vi "test(Subvi).vi"(6 "Frequency(Hz)":dbl, 8 "Amplitude(Vpeak)":dbl, 9 "Pulse length(sec)":dbl, 10 "Delay time.A.1(sec)":dbl, 11 "Sampling frequency(Hz)":dbl) -> ()   [LabVIEW 2017]
uses:
  <vilib>/Analysis/3filter.llb/Filter Passband Type.ctl
  <vilib>/Analysis/4window.llb/windowTd.ctl
  <vilib>/measure/maspectr.llb/FFT Spectrum (Real-Im) for 1 Chan.vi
  <vilib>/Analysis/3filter.llb/FIR Windowed Filter (DBL).vi
  <vilib>/Analysis/NI_AALBase.lvlib
  <vilib>/measure/NI_MAPro.lvlib
  <vilib>/Analysis/NI_AALPro.lvlib
panel:
  out "웨이브폼 그래프 7":waveform(dbl)(graph)
  out "웨이브폼 그래프 6":waveform(dbl)(graph)
  out "웨이브폼 그래프 3":dbl[](graph)
  out "크기":i32
  in  "Carrier Frequency(Hz)":dbl
  out "Delay SIG.A.1":dbl[](array[numeric])
  out "Pulse SIG":dbl[](array[numeric])
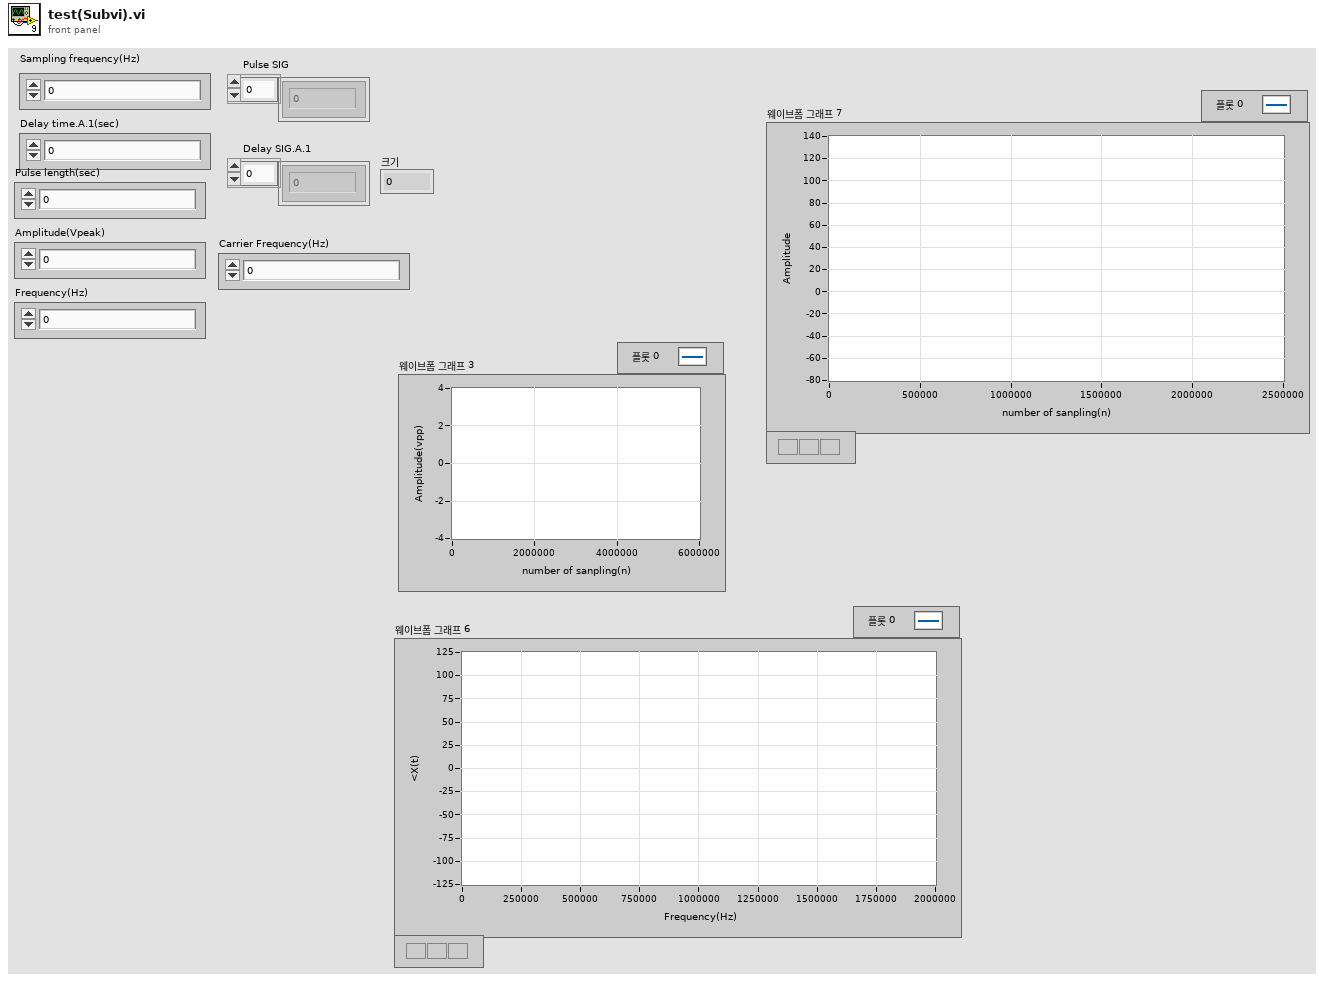
[diagram p1: front panel]
types:
  T1 = typedef "NI_AALBase.lvlib/Filter Passband Type.ctl" = enum32{"Lowpass", "Highpass", "Bandpass", "Bandstop"}
  T2 = cluster{"f0":dbl, "df":dbl, "imaginary part":dbl[]}
  T3 = typedef "NI_AALPro.lvlib/windowTd.ctl" = u32
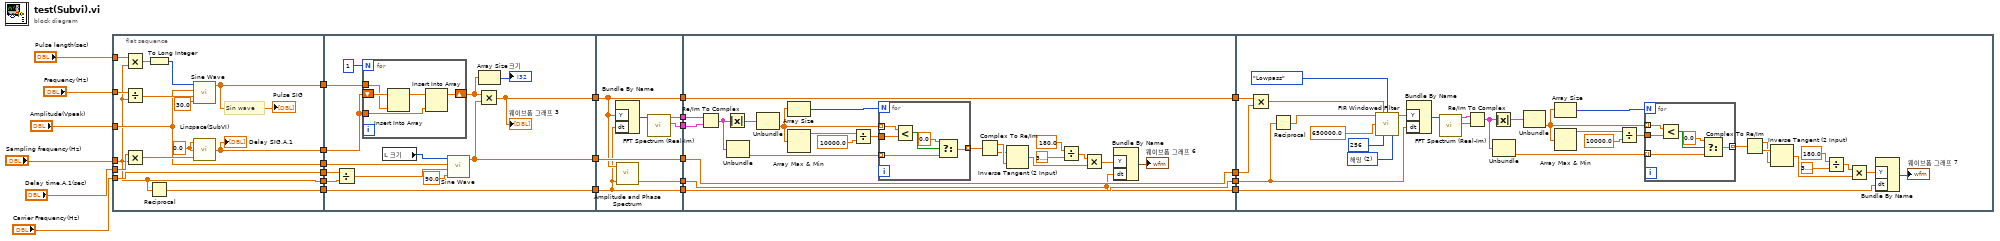
[diagram p0: block diagram]
diagram:
  n1 = flat-sequence {
    tunnel: "Frequency(Hz)" -> [w37]
    tunnel: "Amplitude(Vpeak)" -> [w28]
    tunnel: "Pulse length(sec)" -> [w36]
    tunnel: "Sampling frequency(Hz)" -> [w26]
    tunnel: "Delay time.A.1(sec)" -> [w35]
    tunnel: [w33] -> w20
    tunnel: [w34] -> w19
    tunnel: [w32] -> w18
    tunnel: [w28] -> w17
    tunnel: "Carrier Frequency(Hz)" -> [w27]
    tunnel: [w27] -> w15
    tunnel: [w26] -> w14
    tunnel: w20 -> [w53]
    tunnel: w19 -> [w52]
    tunnel: w18 -> [w43]
    tunnel: w17 -> [w50]
    tunnel: w15 -> [w46]
    tunnel: w14 -> [w45]
    tunnel: [w43] -> w13
    tunnel: [w42] -> w12
    tunnel: [w41] -> w8
    tunnel: w13 -> [w60]
    tunnel: w12 -> [w61]
    tunnel: [w65] -> w11
    tunnel: [w64] -> w10
    tunnel: [w63] -> w9
    tunnel: w8 -> [w62]
    tunnel: [w62] -> w7
    tunnel: [w61] -> w6
    tunnel: [w60] -> w3
    tunnel: w11 -> [w81]
    tunnel: w10 -> [w80]
    tunnel: w9 -> [w72]
    tunnel: w7 -> [w74]
    tunnel: w6 -> [w75]
    tunnel: [w75] -> w5
    tunnel: [w74] -> w4
    tunnel: w3 -> [w73]
    tunnel: [w73] -> w2
    tunnel: [w72] -> w1
    tunnel: w5 -> [w126]
    tunnel: w4 -> [w125]
    tunnel: w2 -> [w98]
    tunnel: w1 -> [w109]
    frame #0 {
      w38 = 0.0 ("frequency")
      # "Sin wave"
      n2 = Multiply(x=w36, y=w26) -> (x*y=w40:dbl)
      n3 = Divide(x=w37, y=w26) -> (x/y=w29:dbl)
      n4 = Multiply(x=w35, y=w26) -> (x*y=w39:dbl)
      n5 = To Long Integer(number=w40) -> (32bit integer=w30:i32)
      n6 = Reciprocal(x=w26) -> (1/x=w32:dbl)
      n7 = call <vilib>:"Sine Wave.vi"("samples"=w30, "amplitude"=w28, "frequency"=w29, "phase in"=30.0) -> ("sine wave"=w33:dbl[])  [unwired: 1 in, 2 out]
      "Pulse SIG" <- w33
      n8 = call "Linspace(SubVI).vi"("NumElements"=w39, "End"=w38, "Start"=w38) -> ("Array"=w34:dbl[])
      "Delay SIG.A.1" <- w34
    }
    frame #1 {
      n9 = Divide(x=w46, y=w45) -> (x/y=w47:dbl)
      n10 = for {
        N: 1 -> [_]
        shift-right: [w55] -> w44
        shift-left: w52 -> [w59]
        tunnel: w53 -> [w58]
        tunnel: w52 -> [w56]
        n11 = Insert Into Array(array=w59, new element=w58) -> (w57:dbl[])  [unwired: 1 in]
        n12 = Insert Into Array(array=w57, new element=w56) -> (w55:dbl[])  [unwired: 1 in]
      }
      n13 = local read "크기"() -> (w48:i32)
      n14 = call <vilib>:"Sine Wave.vi"("samples"=w48, "amplitude"=w50, "frequency"=w47, "phase in"=90.0) -> ("sine wave"=w41:dbl[])  [unwired: 1 in, 2 out]
      n15 = Multiply(x=w44, y=w41) -> (x*y=w42:dbl[])
      "웨이브폼 그래프 3" <- w42
      n16 = Array Size(array=w44) -> (size(s)=→"크기":i32)
    }
    frame #2 {
      n17 = Bundle By Name("Y"=w61, "dt"=w60) -> (w66:waveform(dbl))  [unwired: 1 in]
      n18 = call <vilib>:"Amplitude and Phase Spectrum.vi"("dt"=w60, "Signal (V)"=w61) -> ("df"=w63:dbl)  [unwired: 1 in, 2 out]
      n19 = call-poly <vilib>:"FFT Spectrum (Real-Im).vi"("time signal"=w66) -> ("imaginary part"=w64:T2, "real part"=w65:cluster{"f0":dbl, "df":dbl, "real part":dbl[]})  [unwired: 6 in, 3 out]
    }
    frame #3 {
      n20 = Re/Im To Complex(1:w80, 2:w81) -> (0:w83:cluster{"f0":cdb, "df":cdb, cdb[]})
      n21 = Absolute Value(x=w83) -> (abs(x)=w87:cluster{"f0":dbl, "df":dbl, dbl[]})
      n22 = Unbundle(w83) -> (w82:cdb[])  [unwired: 2 out]
      n23 = Unbundle(w87) -> (w84:dbl[])  [unwired: 2 out]
      n24 = Array Size(array=w84) -> (size(s)=w86:i32)
      n25 = Array Max & Min(array=w84) -> (max value=w89:dbl)  [unwired: 3 out]
      n26 = Divide(x=w89, y=10000.0) -> (x/y=w85:dbl)
      n27 = for {
        N: w86 -> [_]
        tunnel: w85 -> [w95]
        tunnel: w84 -> [w92] mode=indexing
        tunnel: [w91] -> w79 mode=indexing
        tunnel: w82 -> [w90] mode=indexing
        n28 = Less?(x=w92, y=w95) -> (x < y?=w94:bool)
        n29 = Select(t=0.0, s=w94, f=w90) -> (s? t:f=w91:cdb)
      }
      n30 = Complex To Re/Im(x + iy=w79) -> (x=w78:dbl[], y=w77:dbl[])
      n31 = Inverse Tangent (2 Input)(1:w78, 2:w77) -> (0:w69:dbl[])
      n32 = Divide(x=180.0, y=3.141592653589793) -> (x/y=w68:dbl)
      n33 = Multiply(x=w68, y=w69) -> (x*y=w67:dbl[])
      n34 = Bundle By Name("Y"=w67, "dt"=w72) -> (→"웨이브폼 그래프 6":waveform(dbl))  [unwired: 1 in]
    }
    frame #4 {
      w99 = T3 2 items=["사각형"=0, "해닝"=1, "해밍"=2, "블랙맨-해리스"=3, "정밀한 블랙맨"=4, "블랙맨"=5, "플랫 탑"=6, "4항 블랙맨-해리스 "=7, "7항 블랙맨-해리스"=8, "낮은 사이드로브"=9, "블랙맨 누탈"=11, "삼각형"=30, "바틀렛-해닝"=31, "보먼"=32, "파젠"=33, "웰치"=34, "카이저"=60, "돌프-체비셰프"=61, "가우스"=62] ("window")
      n35 = Multiply(x=w126, y=w125) -> (x*y=w102:dbl[])
      n36 = Reciprocal(x=w98) -> (1/x=w97:dbl)
      n37 = call-poly <vilib>:"FIR Windowed Filter.vi"("sampling freq: fs"=w97, "X"=w102, "filter type"=Filter_Passband_Type."Lowpass", "low cutoff freq: fl"=650000.0 ("high cutoff freq: fh"), "taps"=256 ("order"), "window"=w99) -> ("Filtered X"=w100:dbl[])  [unwired: 8 in, 1 out]
      n38 = Bundle By Name("Y"=w100, "dt"=w98) -> (w124:waveform(dbl))  [unwired: 1 in]
      n39 = call-poly <vilib>:"FFT Spectrum (Real-Im).vi"("time signal"=w124) -> ("imaginary part"=w110:T2, "real part"=w111:cluster{"f0":dbl, "df":dbl, "real part":dbl[]})  [unwired: 6 in, 3 out]
      n40 = Re/Im To Complex(1:w110, 2:w111) -> (0:w118:cluster{"f0":cdb, "df":cdb, cdb[]})
      n41 = Absolute Value(x=w118) -> (abs(x)=w114:cluster{"f0":dbl, "df":dbl, dbl[]})
      n42 = Unbundle(w118) -> (w119:cdb[])  [unwired: 2 out]
      n43 = Unbundle(w114) -> (w117:dbl[])  [unwired: 2 out]
      n44 = Array Size(array=w117) -> (size(s)=w115:i32)
      n45 = Array Max & Min(array=w117) -> (max value=w113:dbl)  [unwired: 3 out]
      n46 = Divide(x=w113, y=10000.0) -> (x/y=w116:dbl)
      n47 = for {
        N: w115 -> [_]
        tunnel: w116 -> [w132]
        tunnel: w117 -> [w129] mode=indexing
        tunnel: [w128] -> w120 mode=indexing
        tunnel: w119 -> [w127] mode=indexing
        n48 = Less?(x=w129, y=w132) -> (x < y?=w131:bool)
        n49 = Select(t=0.0, s=w131, f=w127) -> (s? t:f=w128:cdb)
      }
      n50 = Complex To Re/Im(x + iy=w120) -> (x=w121:dbl[], y=w122:dbl[])
      n51 = Inverse Tangent (2 Input)(1:w121, 2:w122) -> (0:w105:dbl[])
      n52 = Divide(x=180.0, y=3.141592653589793) -> (x/y=w106:dbl)
      n53 = Multiply(x=w106, y=w105) -> (x*y=w104:dbl[])
      n54 = Bundle By Name("Y"=w104, "dt"=w109) -> (→"웨이브폼 그래프 7":waveform(dbl))  [unwired: 1 in]
    }
  }
